vi "test12.vi"() -> ()   [LabVIEW 2016]
uses:
  <vilib>/Analysis/NI_AALBase.lvlib
panel:
  out "variance":dbl format="%0.2f"
  out "standard deviation":dbl format="%0.2f"
  out "mean":dbl format="%0.2f"
  in  "Array 2":dbl[][][](array[numeric])
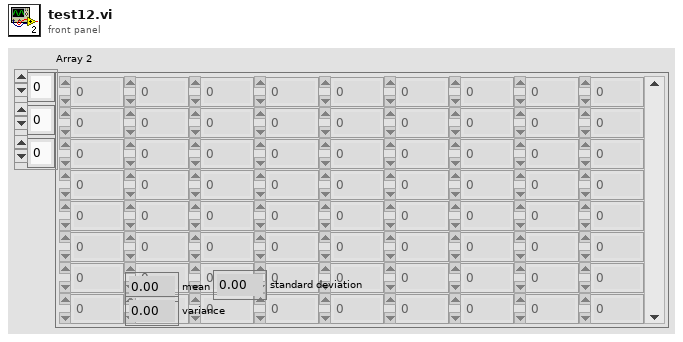
[diagram p1: front panel]
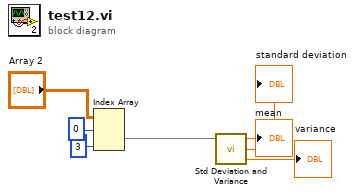
[diagram p0: block diagram]
diagram:
  n1 = Index Array(array="Array 2", index (dim 0)=0 ("index (page)"), index (dim 2)=3 ("disabled index (col)")) -> (element=w4:dbl[])  [unwired: 1 in]
  n2 = call <vilib>:"Std Deviation and Variance.vi"("X"=w4) -> ("mean"=→"mean":dbl, "standard deviation"=→"standard deviation":dbl, "variance"=→"variance":dbl)  [unwired: 1 in]
